vi "Clear_Actor_Test.vi"(8 "error in (no error)":errorcluster caption="entrée d'erreur (pas d'erreur)", 11 "Test (Default) en entrée":refnum<class "Actor Test (Default).lvclass">) -> (0 "error out":errorcluster caption="sortie d'erreur", 3 "Test (Default) en sortie":refnum<class "Actor Test (Default).lvclass">)   [LabVIEW 2020, in "Library Core.lvlib" / "Actor Test (Default).lvclass"]
uses:
  Actor Test (Default).lvclass
  Actor Test (Default).lvclass/Actor Test (Default).ctl
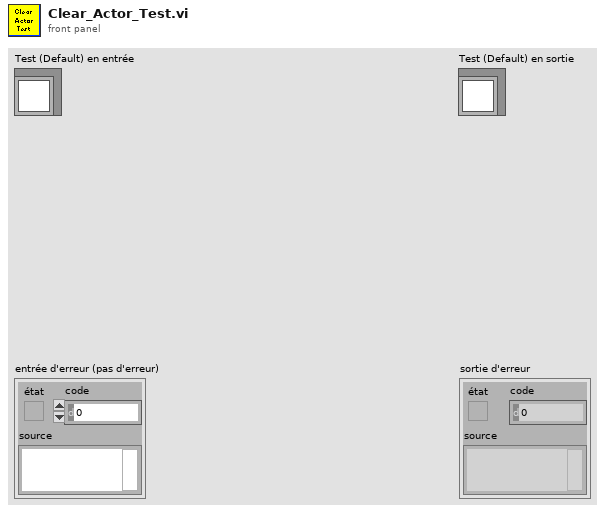
[diagram p1: front panel]
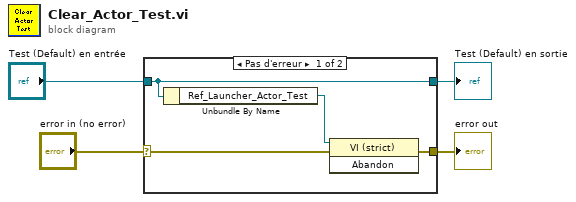
[diagram p0: block diagram]
diagram:
  n1 = case shown="Pas d'erreur" "error in (no error)" {
    selector: "error in (no error)" -> [w7 w10]
    tunnel: [w6 w10] -> w3
    tunnel: [w8 w9] -> w1
    tunnel: "Test (Default) en entrée" -> [w8 w9]
    frame No Error {
      n2 = Unbundle By Name(w8) -> ("Ref_Launcher_Actor_Test"=w5:refnum<vi>)
      n3 = invoke class="VI (strict)" method="Abandon"(reference=w5, error in=w7) -> (error out=w6:errorcluster)  [unwired: 1 in, 2 out]
    }
    frame Error {
    }
  }
  "error out" <- w3
  "Test (Default) en sortie" <- w1
